vi "Destroy.vi"(8 "error in (no error)":errorcluster, 11 "String In":refnum<class "String.lvclass">) -> (0 "error out":errorcluster, 3 "String Out":refnum<class "String.lvclass">)   [LabVIEW 2015, in "Front Panel Publisher.lvlib" / "String.lvclass"]
uses:
  String.lvclass
  Control_class/Control.lvclass
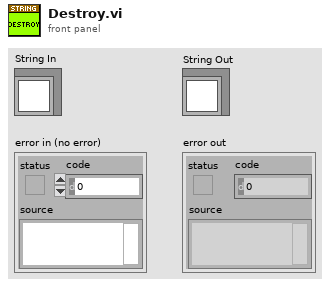
[diagram p1: front panel]
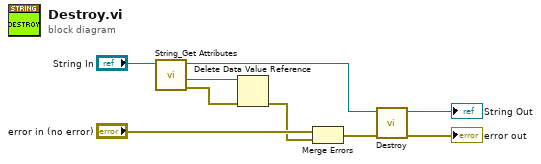
[diagram p0: block diagram]
diagram:
  n1 = call "String_Get Attributes.vi"("String In"="String In") -> ("error out"=w8:errorcluster, "DataRef"=w7:refnum<data-value>, "String Out"=w4:refnum<class "String.lvclass">)  [unwired: 7 in, 1 out]
  n2 = Delete Data Value Reference(data value reference=w7, error in=w8) -> (error out=w5:errorcluster)  [unwired: 1 out]
  n3 = Merge Errors("error in (no error)", w5) -> (w1:errorcluster)
  n4 = call-parent "Destroy.vi"("error in (no error)"=w1, "Control In"=w4) -> ("error out"=→"error out":errorcluster, "Control Out"=→"String Out":refnum<class "String.lvclass">)  [unwired: 8 in]
